vi "act-0010-2-en.vi"() -> ()   [LabVIEW 2010]
panel:
  in  "Choix (K ou F ou C)":string
  out "affichage":dbl caption="Temp simulée en °F"
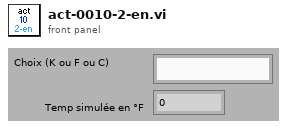
[diagram p1: front panel]
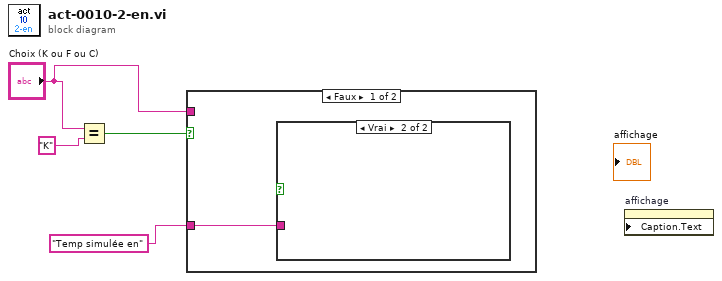
[diagram p0: block diagram]
diagram:
  n1 = Equal?(x="Choix (K ou F ou C)", y="K") -> (x = y?=w3:bool)
  n2 = case shown="Faux" w3 {
    tunnel: "Temp simulée en" -> [w5 _]
    tunnel: "Choix (K ou F ou C)" -> [_ _]
    frame False {
      n3 = case shown="Vrai" {
        selector: _ -> [_ _]
        tunnel: w5 -> [_ _]
        frame False {
        }
        frame True {
        }
      }
    }
    frame True {
    }
  }
  n4 = property on="affichage" class="NumDig (strict)" props=["Caption", "Text"]() -> ()  [unwired: 3 in, 2 out]
